vi "Set Acceleration.vi"(8 "error in (no error)":errorcluster, 9 "Y Axis":u16, 10 "X Axis":u16, 11 "2-Axis Stage in":refnum<class "Sync 2-Axis Stage Controller.lvclass">) -> (0 "error out":errorcluster, 3 "2-Axis Stage out":refnum<class "Sync 2-Axis Stage Controller.lvclass">)   [LabVIEW 2022 SP3, in "Sync 2-Axis Stage Controller.lvclass"]
uses:
  Sync 2-Axis Stage Controller.lvclass
  Axis Objects/iMotion Controller/iMotion Controller.lvclass
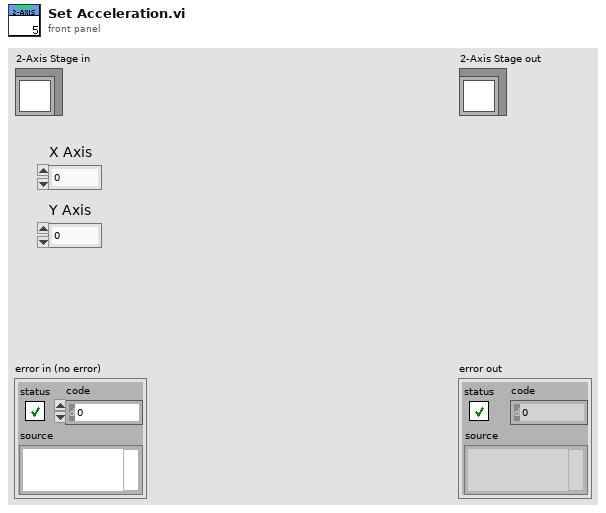
[diagram p1: front panel]
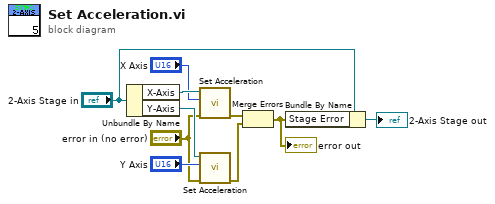
[diagram p0: block diagram]
diagram:
  n1 = Unbundle By Name("2-Axis Stage in") -> ("X-Axis"=w9:refnum<class "iMotion Controller.lvclass">, "Y-Axis"=w8:refnum<class "iMotion Controller.lvclass">)
  n2 = call-dynamic "Set Acceleration.vi"("error in (no error)"="error in (no error)", "Acceleration"="X Axis", "iMotion Controller in"=w9) -> ("error out"=w5:errorcluster)  [unwired: 7 in, 1 out]
  n3 = call-dynamic "Set Acceleration.vi"("error in (no error)"="error in (no error)", "Acceleration"="Y Axis", "iMotion Controller in"=w8) -> ("error out"=w4:errorcluster)  [unwired: 7 in, 1 out]
  n4 = Merge Errors(w5, w4) -> (w1:errorcluster)
  "error out" <- w1
  n5 = Bundle By Name(cluster="2-Axis Stage in", "Stage Error"=w1) -> (→"2-Axis Stage out":refnum<class "Sync 2-Axis Stage Controller.lvclass">)
